vi "Volmeter Error Correction.vi"(4 "Относительная погрешность Rвн, %":dbl, 5 "Rвх вольтметра, Ом":dbl, 6 "Rвн source, Om":dbl, 7 "Показания вольтметра, В":dbl) -> (0 "Неисключенная методическа погрешность, В":dbl, 1 "Исправленные показания,В":dbl, 2 "Поправка, В":dbl, 3 "Методическая погрешность,В":dbl)   [LabVIEW 2013]
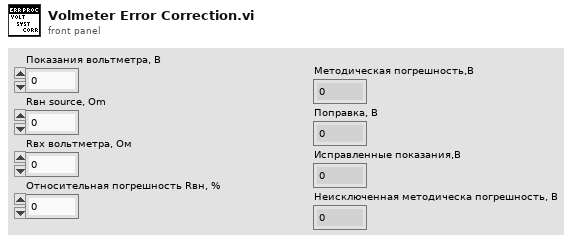
[diagram p1: front panel]
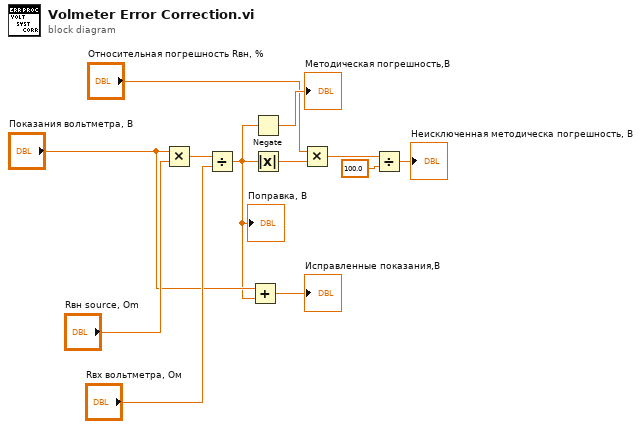
[diagram p0: block diagram]
diagram:
  n1 = Multiply(x="Показания вольтметра, В", y="Rвн source, Om") -> (x*y=w11:dbl)
  n2 = Divide(x=w11, y="Rвх вольтметра, Ом") -> (x/y=w1:dbl)
  "Поправка, В" <- w1
  n3 = Add(x="Показания вольтметра, В", y=w1) -> (x+y=→"Исправленные показания,В":dbl)
  n4 = Negate(x=w1) -> (-x=→"Методическая погрешность,В":dbl)
  n5 = Absolute Value(x=w1) -> (abs(x)=w5:dbl)
  n6 = Multiply(x="Относительная погрешность Rвн, %", y=w5) -> (x*y=w3:dbl)
  n7 = Divide(x=w3, y=100.0) -> (x/y=→"Неисключенная методическа погрешность, В":dbl)
